vi "svx_Polar_Property_Change.vi"(0 "Property Name":string, 1 "Display State In":T2={"Property Name"=[], "Container bounds"={"Width"=550, "Height"=250}, "Scale range"={"Maximum"=1.0, "Increment"=1.0}, "PointIdx"=0, "Marker list"=[], "Color settings"={"Arrow color"=16860, "Magnitude major grid"=13816530, "Magnitude minor grid"=16777216, "Phase grid"=13816530, "Phase scale marker text"=0}, "Magnitude scale name"="Magnitude", "Magnitude scale format string"="%#.2e", "MagnitudeScale:Visible"=TRUE, "MagnitudeScaleLabel:Visible"=TRUE, "PhaseScale:Visible"=TRUE, "Marker:Visible"=TRUE, "Cursor:Visible"=FALSE, "CursorName:Visible"=TRUE, "Autoscale"=TRUE, "Marker color"=16860, "Line color"=16711680, "Cursor color"=16711680, "Magnitude scale marker color"=0, "Plot.Line Style"=0, "Plot.Line Width"=0, "Plot.Point Style"=0, "Cursor.Line Style"=0, "Cursor.Line Width"=0, "Cursor.Point Style"=0, "Cursor.Style"=4, "Marker.Point Style"=2, "Point/fill color"=16711680, "Background color"=16777225, "Cursor name"="", "Cursor Release"=refnum, "Scale Range Change"=refnum, "data size(s)"=[], "Selectors:Visible"=TRUE, "Selector:ring Strings"={"Selector:Custom Strings"=FALSE, "Selector:Row Strings []"=[], "Selector:Column Strings []"=[], "User:Row Strings []"=[], "User:Column Strings []"=[]}, "Lock Cursor Info Position"=FALSE, "CursLoc"={"magnitude"=0.0, "phase"=0.0, "time/rev/RPM"=0.0}, "Plot Area:Position"={"Left"=0, "Top"=0}, "Plot Area:Size"={"Width"=0, "Height"=0}, "Marker.Style"=0, "Indication Arcs"=[], "Arc.Selector"=0, "customized marker"=[], "tree Width"=0, " Parents Tags"=[], "Children Tags"=[], "open?"=[], "index"=[{"row index"=0, "column index"=0}], "Label"="", "custom strings changed"=FALSE, "Owning VI"=refnum, "Legend BG color"=16777225, "Legend font color"=0, "column Width"=203, "attribute"=variant} caption="State", 2 "data":T1, 5 "operation in":T5[](array[typedef]), 6 "Plot Legend":refnum<vi>, 7 "z scale graph":refnum<vi>, 8 "Polar Plot ref in":refnum<vi>, 9 "Cursor Info":refnum<vi>, 10 "Container Refnum":refnum<vi>) -> (15 "Display State Out":T2={"Property Name"=[], "Container bounds"={"Width"=550, "Height"=250}, "Scale range"={"Maximum"=1.0, "Increment"=1.0}, "PointIdx"=0, "Marker list"=[], "Color settings"={"Arrow color"=16860, "Magnitude major grid"=13816530, "Magnitude minor grid"=16777216, "Phase grid"=13816530, "Phase scale marker text"=0}, "Magnitude scale name"="Magnitude", "Magnitude scale format string"="%#.2e", "MagnitudeScale:Visible"=TRUE, "MagnitudeScaleLabel:Visible"=TRUE, "PhaseScale:Visible"=TRUE, "Marker:Visible"=TRUE, "Cursor:Visible"=FALSE, "CursorName:Visible"=TRUE, "Autoscale"=TRUE, "Marker color"=16860, "Line color"=16711680, "Cursor color"=16711680, "Magnitude scale marker color"=0, "Plot.Line Style"=0, "Plot.Line Width"=0, "Plot.Point Style"=0, "Cursor.Line Style"=0, "Cursor.Line Width"=0, "Cursor.Point Style"=0, "Cursor.Style"=4, "Marker.Point Style"=2, "Point/fill color"=16711680, "Background color"=16777225, "Cursor name"="", "Cursor Release"=refnum, "Scale Range Change"=refnum, "data size(s)"=[], "Selectors:Visible"=TRUE, "Selector:ring Strings"={"Selector:Custom Strings"=FALSE, "Selector:Row Strings []"=[], "Selector:Column Strings []"=[], "User:Row Strings []"=[], "User:Column Strings []"=[]}, "Lock Cursor Info Position"=FALSE, "CursLoc"={"magnitude"=0.0, "phase"=0.0, "time/rev/RPM"=0.0}, "Plot Area:Position"={"Left"=0, "Top"=0}, "Plot Area:Size"={"Width"=0, "Height"=0}, "Marker.Style"=0, "Indication Arcs"=[], "Arc.Selector"=0, "customized marker"=[], "tree Width"=0, " Parents Tags"=[], "Children Tags"=[], "open?"=[], "index"=[{"row index"=0, "column index"=0}], "Label"="", "custom strings changed"=FALSE, "Owning VI"=refnum, "Legend BG color"=16777225, "Legend font color"=0, "column Width"=203, "attribute"=variant} caption="State", 19 "operation out":T5[](array[typedef]))   [LabVIEW 2017, in "SVX Polar Plot.xctl"]
uses:
  <vilib>/addons/_XControls/Polar Plot/SVX Polar Plot.xctl
  <vilib>/addons/_XControls/Polar Plot/subVIs/svx_Polar_Plot_Internal_State.ctl
  <vilib>/addons/_XControls/Polar Plot/subVIs/svx_Polar_Indication_Arcs.ctl
  <vilib>/addons/_XControls/Polar Plot/subVIs/svx_Polar_Customized_Markers.ctl
  <vilib>/addons/_XControls/Polar Plot/subVIs/svx_Polar_Core_States.ctl
  <vilib>/Utility/miscctls.llb/LVAnnotationListTypeDef.ctl
  <vilib>/Utility/miscctls.llb/LVBoundsTypeDef.ctl
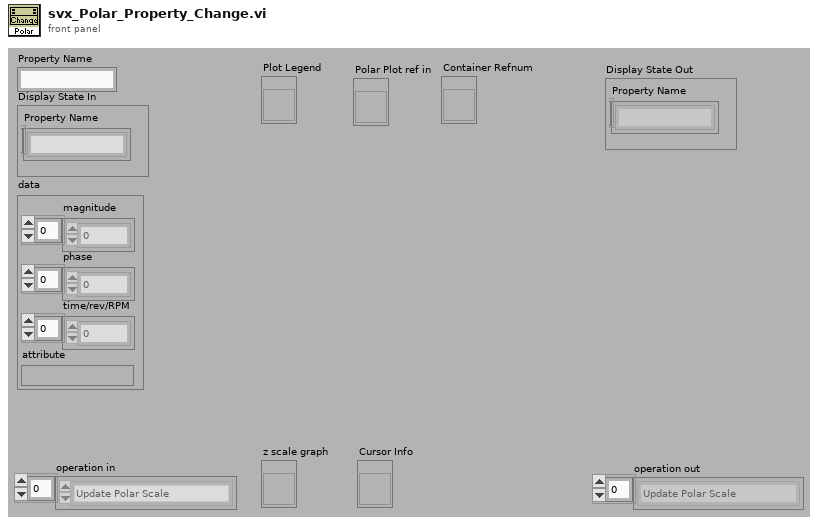
[diagram p1: front panel]
types:
  T1 = cluster{"magnitude":dbl[], "phase":dbl[], "time/rev/RPM":dbl[], "attribute":variant}
  T2 = typedef "SVX Polar Plot.xctl/svx_Polar_Plot_Internal_State.ctl" = cluster{"Property Name":string[], "Container bounds":cluster{"Width":u32, "Height":u32}, "Scale range":cluster{"Maximum":dbl, "Increment":dbl}, "PointIdx":i32, "Marker list":cluster{"Name":string, "Color":u32, "Style":u8, "Point Style":u8, "Name Visible":bool, "Allow Drag":bool, "Annotation Mode":u32, "Plot":i32, "Index":i32, "Position":cluster{"X":dbl, "Y":dbl}, "X Scale":u32, "Y Scale":u32, "Show Arrow":bool, "Lock Name":bool, "Plot Area":i32, "Label Offset":cluster{"X":dbl, "Y":dbl}}[], "Color settings":cluster{"Arrow color":u32, "Magnitude major grid":u32, "Magnitude minor grid":u32, "Phase grid":u32, "Phase scale marker text":u32}, "Magnitude scale name":string, "Magnitude scale format string":string, "MagnitudeScale:Visible":bool, "MagnitudeScaleLabel:Visible":bool, "PhaseScale:Visible":bool, "Marker:Visible":bool, "Cursor:Visible":bool, "CursorName:Visible":bool, "Autoscale":bool, "Marker color":u32, "Line color":u32, "Cursor color":u32, "Magnitude scale marker color":u32, "Plot.Line Style":i32, "Plot.Line Width":i32, "Plot.Point Style":i32, "Cursor.Line Style":i32, "Cursor.Line Width":i32, "Cursor.Point Style":i32, "Cursor.Style":i32, "Marker.Point Style":i32, "Point/fill color":u32, "Background color":u32, "Cursor name":string, "Cursor Release":refnum<user-event>, "Scale Range Change":refnum<user-event>, "data size(s)":i32[], "Selectors:Visible":bool, "Selector:ring Strings":cluster{"Selector:Custom Strings":bool, "Selector:Row Strings []":string[], "Selector:Column Strings []":string[], "User:Row Strings []":string[], "User:Column Strings []":string[]}, "Lock Cursor Info Position":bool, "CursLoc":cluster{"magnitude":dbl, "phase":dbl, "time/rev/RPM":dbl}, "Plot Area:Position":cluster{"Left":i32, "Top":i32}, "Plot Area:Size":cluster{"Width":u32, "Height":u32}, "Marker.Style":i32, "Indication Arcs":T3, "Arc.Selector":u16, "customized marker":T4, "tree Width":u32, " Parents Tags":string[], "Children Tags":string[], "open?":bool[], "index":cluster{"row index":i32, "column index":i32}[], "Label":string, "custom strings changed":bool, "Owning VI":refnum<vi>, "Legend BG color":u32, "Legend font color":u32, "column Width":u32, "attribute":variant}
  T3 = typedef "SVX Polar Plot.xctl/svx_Polar_Indication_Arcs.ctl" = cluster{"Name":string, "Start radius":dbl, "End radius":dbl, "Line Style":i32, "Line Width":i32, "Border color":u32, "Fill color":u32, "Start angle":i16, "End angle":i16, "Visible":bool}[]
  T4 = typedef "SVX Polar Plot.xctl/svx_Polar_Customized_Markers.ctl" = cluster{"Name":string, "Color":u32, "Style":u8, "Point Style":u8, "Name Visible":bool, "Allow Drag":bool, "Annotation Mode":u32, "Plot":i32, "Index":i32, "Position":cluster{"Magnitude":dbl, "Phase":dbl}, "X Scale":u32, "Y Scale":u32, "Show Arrow":bool, "Lock Name":bool, "Plot Area":i32, "Label Offset":cluster{"Magnitude":dbl, "Phase":dbl}}[]
  T5 = typedef "SVX Polar Plot.xctl/svx_Polar_Core_States.ctl" = enum16{"Update Polar Scale", "Cursor Release", "Autoscale", "Update Annotation", "Force Update Polar Scale", "Update Data", "Update Tree String", "Update Tree Checkbox", "Update Tree Opening", "Change Minimum Size"}
  T6 = typedef "LVAnnotationListTypeDef.ctl" = cluster{"Name":string, "Color":u32, "Style":u8, "Point Style":u8, "Name Visible":bool, "Allow Drag":bool, "Annotation Mode":u32, "Plot":i32, "Index":i32, "Position":cluster{"X":dbl, "Y":dbl}, "X Scale":u32, "Y Scale":u32, "Show Arrow":bool, "Lock Name":bool, "Plot Area":i32, "Label Offset":cluster{"X":dbl, "Y":dbl}}[]
  T7 = typedef "LVBoundsTypeDef.ctl" = cluster{"Width":u32, "Height":u32}
  T8 = typedef "LVCursorListTypeDef.ctl" = cluster{"Name":string, "Color":u32, "Style":u8, "Point Style":u8, "Name Visible":bool, "Allow Drag":bool, "Cursor Mode":u32, "Plot":i32, "Index":i32, "Position":cluster{"X":dbl, "Y":dbl}, "X Scale":u32, "Y Scale":u32, "Watch Plots":i32[], "Watch All Plots":bool, "Plot Area":i32, "Label Offset":cluster{"X":dbl, "Y":dbl}}[]
  T9 = cluster{"Name":string, "Color":u32, "Style":u8, "Point Style":u8, "Name Visible":bool, "Allow Drag":bool, "Cursor Mode":u32, "Plot":i32, "Index":i32, "Position":cluster{"X":dbl, "Y":dbl}, "X Scale":u32, "Y Scale":u32, "Watch Plots":i32[], "Watch All Plots":bool, "Plot Area":i32, "Label Offset":cluster{"X":dbl, "Y":dbl}}
  T10 = cluster{"Arrow color":u32, "Magnitude major grid":u32, "Magnitude minor grid":u32, "Phase grid":u32, "Phase scale marker text":u32}
  T11 = cluster{"Name":string, "Color":u32, "Style":u8, "Point Style":u8, "Name Visible":bool, "Allow Drag":bool, "Annotation Mode":u32, "Plot":i32, "Index":i32, "Position":cluster{"X":dbl, "Y":dbl}, "X Scale":u32, "Y Scale":u32, "Show Arrow":bool, "Lock Name":bool, "Plot Area":i32, "Label Offset":cluster{"X":dbl, "Y":dbl}}[]
  T12 = cluster{"Name":string, "Color":u32, "Style":u8, "Point Style":u8, "Name Visible":bool, "Allow Drag":bool, "Annotation Mode":u32, "Plot":i32, "Index":i32, "Position":cluster{"X":dbl, "Y":dbl}, "X Scale":u32, "Y Scale":u32, "Show Arrow":bool, "Lock Name":bool, "Plot Area":i32, "Label Offset":cluster{"X":dbl, "Y":dbl}}
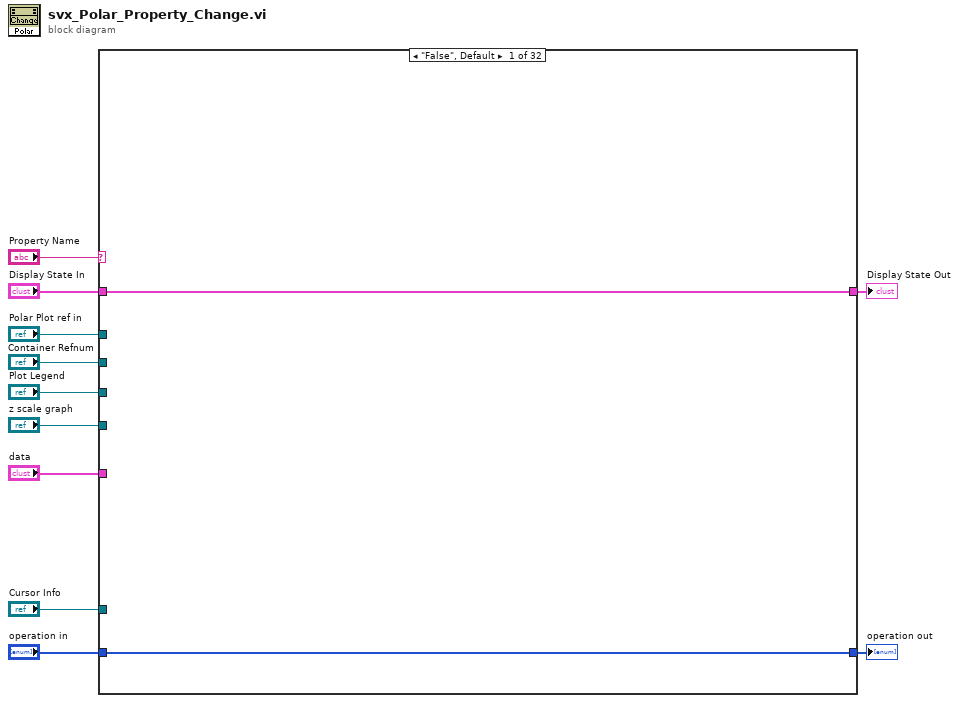
[diagram p0: block diagram]
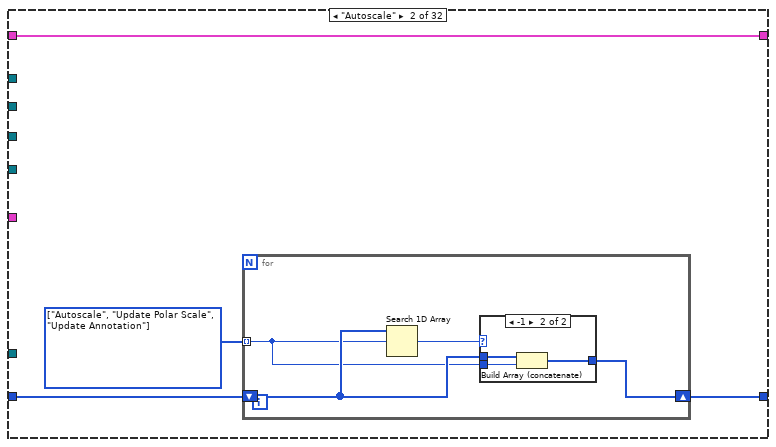
[diagram p2: hidden frame]
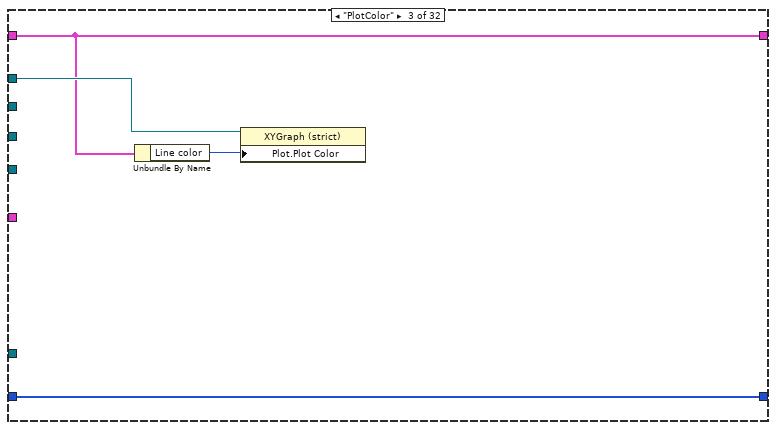
[diagram p4: hidden frame]
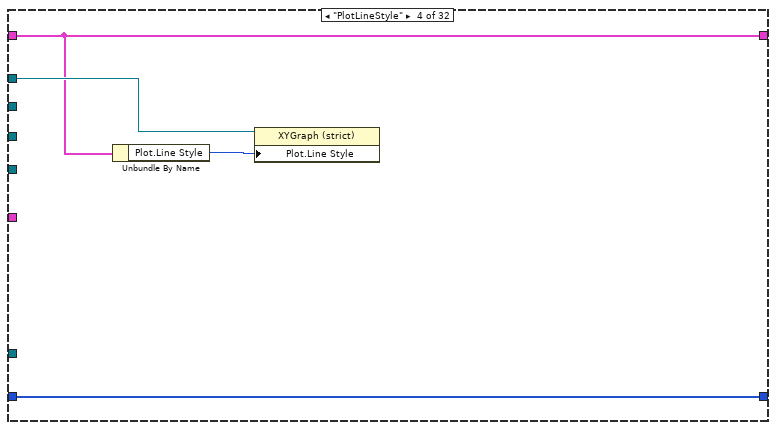
[diagram p5: hidden frame]
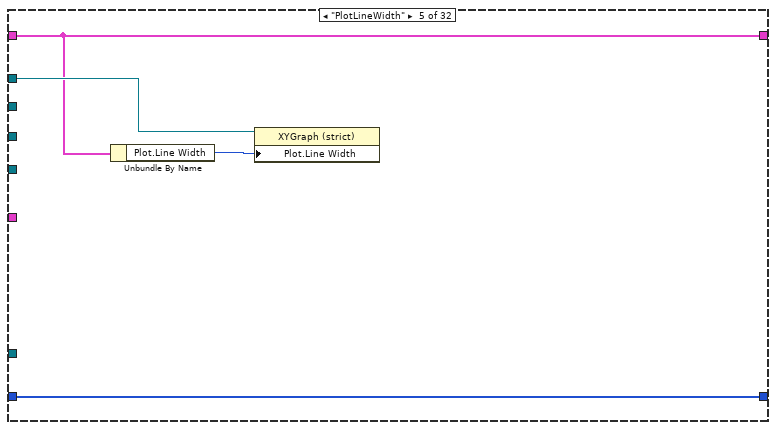
[diagram p6: hidden frame]
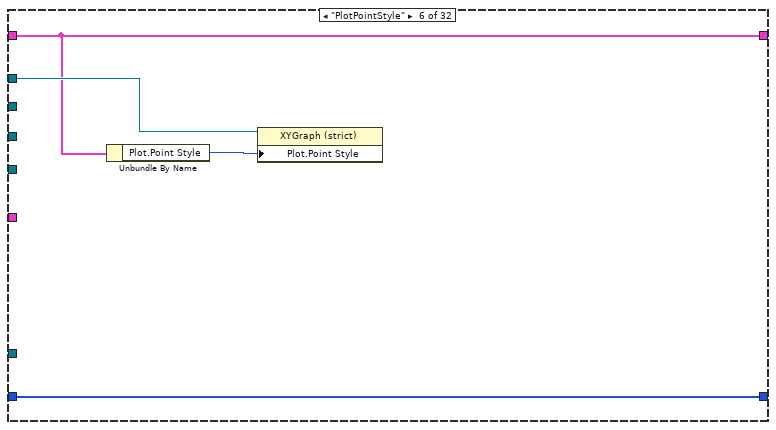
[diagram p7: hidden frame]
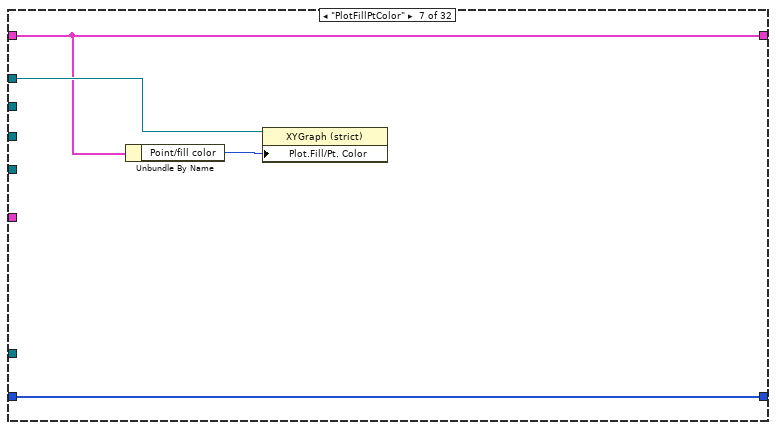
[diagram p8: hidden frame]
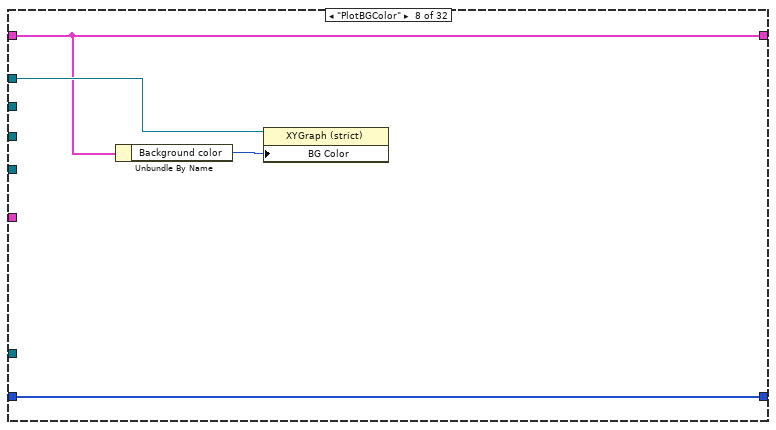
[diagram p9: hidden frame]
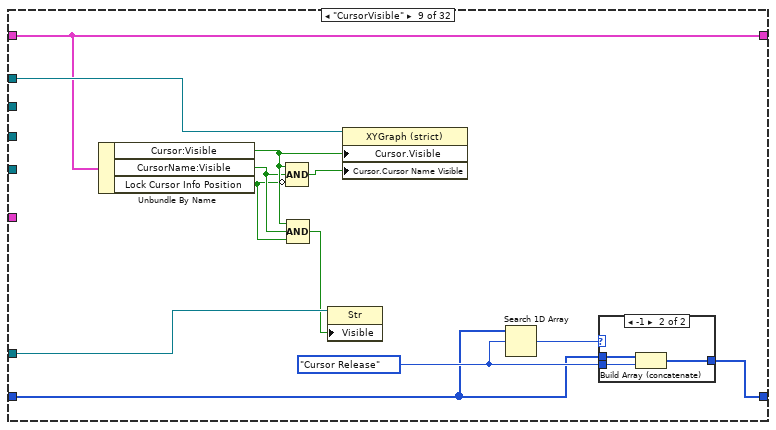
[diagram p10: hidden frame]
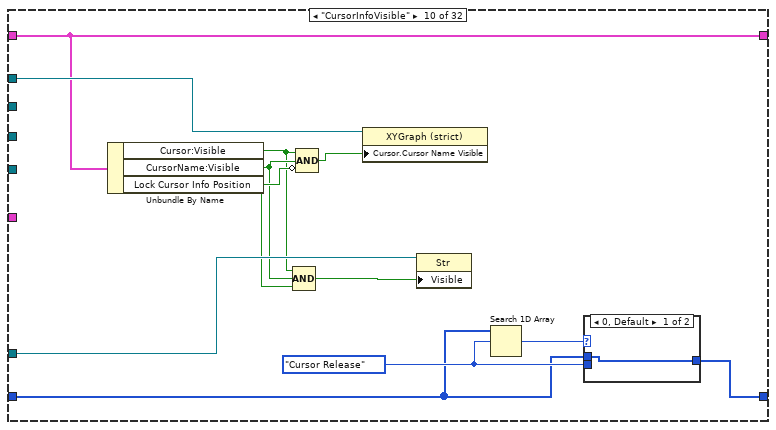
[diagram p12: hidden frame]
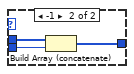
[diagram p13: hidden frame]
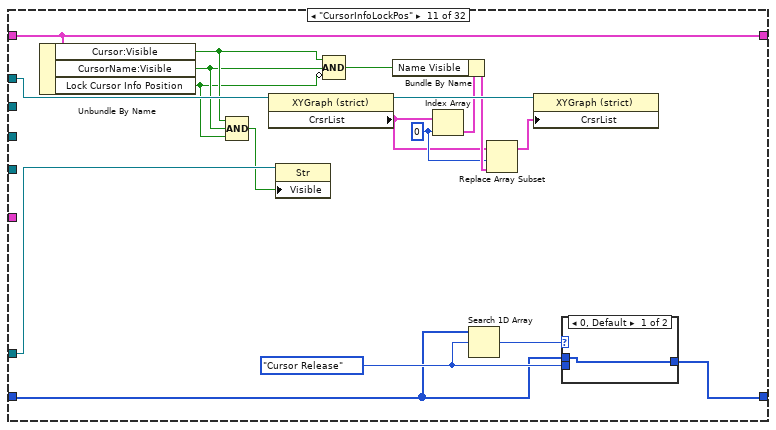
[diagram p14: hidden frame]
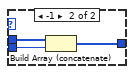
[diagram p15: hidden frame]
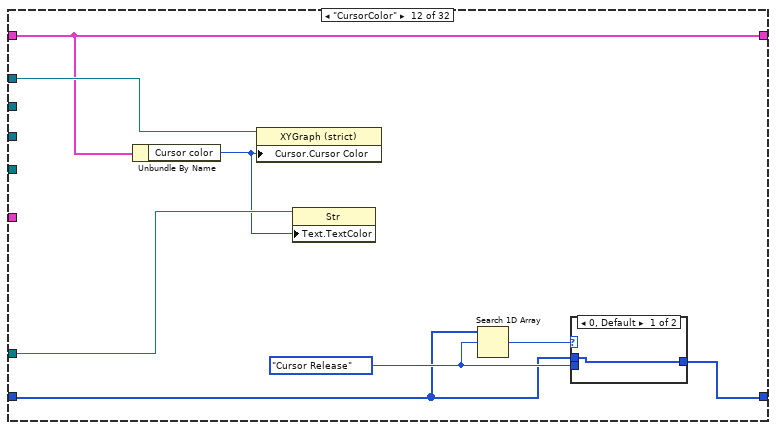
[diagram p16: hidden frame]
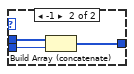
[diagram p17: hidden frame]
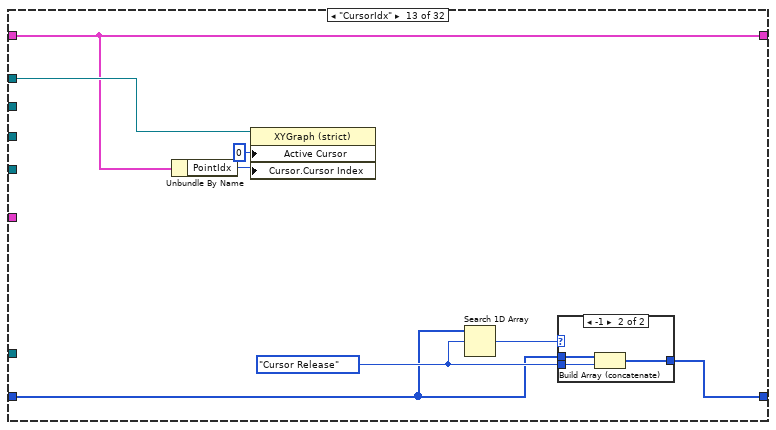
[diagram p18: hidden frame]
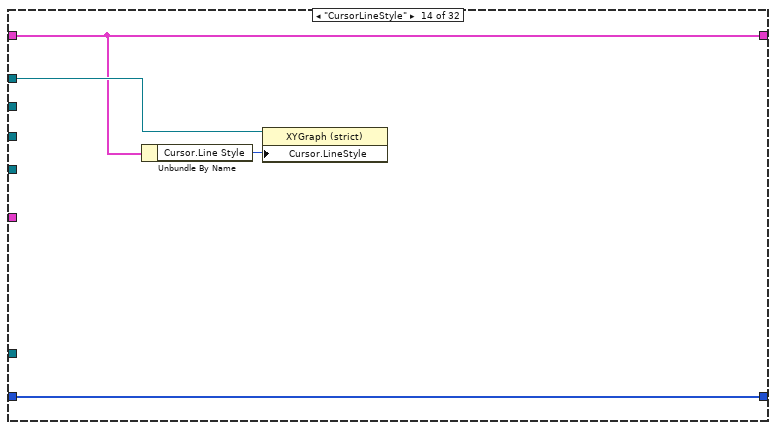
[diagram p20: hidden frame]
diagram:
  n1 = case shown="\"False\", Default" "Property Name" {
    tunnel: "Display State In" -> [w12 w16 w26 w30 w34 w38 w42 w46 w60 w76 w99 w110 w122 w128 w132 w136 w140 w144 w166 w176 w180 w188 w197 w207 w221 w230 w265 w279 w290 w303 w308 w312]
    tunnel: "operation in" -> [w13 w15 w29 w33 w37 w41 w45 w49 w50 w67 w88 w104 w116 w131 w135 w139 w143 w145 w167 w177 w181 w190 w193 w206 w223 w226 w263 w273 w284 w307 _ w315]
    tunnel: [w13 w17 w29 w33 w37 w41 w45 w49 w51 w66 w87 w105 w117 w131 w135 w139 w143 w145 w167 w177 w181 w190 w194 w204 w223 w226 w263 w273 w284 w305 w309 w315] -> w8
    tunnel: "Polar Plot ref in" -> [_ _ w28 w32 w36 w40 w44 w48 w61 w77 w92 w111 w123 w130 w134 w138 w142 w148 w170 _ _ w187 _ w212 w222 w229 w262 w274 w285 w301 _ _]
    tunnel: "z scale graph" -> [_ _ _ _ _ _ _ _ _ _ _ _ _ _ _ _ _ w147 w169 w179 w183 w186 w199 w211 _ w224 _ _ _ w299 _ _]
    tunnel: "data" -> [_ _ _ _ _ _ _ _ _ _ _ _ _ _ _ _ _ _ w165 _ _ _ _ _ _ w228 _ _ _ _ _ _]
    tunnel: [w12 w16 w26 w30 w34 w38 w42 w46 w60 w76 w99 w110 w122 w128 w132 w136 w140 w144 w166 w176 w180 w188 w197 w207 w221 w227 w264 w275 w286 w304 w308 w312] -> w6
    tunnel: "Cursor Info" -> [_ _ _ _ _ _ _ _ w59 w74 w91 w109 _ _ _ _ _ _ _ _ _ _ _ _ _ _ _ _ _ _ _ _]
    tunnel: "Plot Legend" -> [_ _ _ _ _ _ _ _ _ _ _ _ _ _ _ _ _ _ _ _ _ _ _ _ _ _ _ _ _ w300 _ w314]
    tunnel: "Container Refnum" -> [_ _ _ _ _ _ _ _ _ _ _ _ _ _ _ _ _ _ _ _ _ _ _ _ _ _ _ _ _ w302 _ _]
    frame "False", Default {
    }
    frame "Autoscale" {
      w14 = T5[] [enum."Autoscale", enum."Update Polar Scale", enum."Update Annotation"] items=["Update Polar Scale", "Cursor Release", "Autoscale", "Update Annotation", "Force Update Polar Scale", "Update Data", "Update Tree String", "Update Tree Checkbox", "Update Tree Opening", "Change Minimum Size"]
      n2 = for {
        shift-right: [w21] -> w17
        shift-left: w15 -> [w20]
        tunnel: w14 -> [w18] mode=indexing
        n3 = Search 1D Array(1D array=w20, element=w18) -> (index of element=w19:i32)  [unwired: 1 in]
        n4 = case shown="-1" w19 {
          tunnel: [w22 w25] -> w21
          tunnel: w20 -> [w22 w24]
          tunnel: w18 -> [_ w23]
          frame 0, Default {
          }
          frame -1 {
            n5 = Build Array (concatenate)(w24, w23) -> (w25:T5[])
          }
        }
      }
    }
    frame "PlotColor" {
      n6 = Unbundle By Name(w26) -> ("Line color"=w27:u32)
      n7 = property class="XYGraph (strict)"(reference=w28, "Plot.Plot Color"=w27) -> ()  [unwired: 1 in, 2 out]
    }
    frame "PlotLineStyle" {
      n8 = Unbundle By Name(w30) -> ("Plot.Line Style"=w31:i32)
      n9 = property class="XYGraph (strict)"(reference=w32, "Plot.Line Style"=w31) -> ()  [unwired: 1 in, 2 out]
    }
    frame "PlotLineWidth" {
      n10 = Unbundle By Name(w34) -> ("Plot.Line Width"=w35:i32)
      n11 = property class="XYGraph (strict)"(reference=w36, "Plot.Line Width"=w35) -> ()  [unwired: 1 in, 2 out]
    }
    frame "PlotPointStyle" {
      n12 = Unbundle By Name(w38) -> ("Plot.Point Style"=w39:i32)
      n13 = property class="XYGraph (strict)"(reference=w40, "Plot.Point Style"=w39) -> ()  [unwired: 1 in, 2 out]
    }
    frame "PlotFillPtColor" {
      n14 = Unbundle By Name(w42) -> ("Point/fill color"=w43:u32)
      n15 = property class="XYGraph (strict)"(reference=w44, "Plot.Fill/Pt. Color"=w43) -> ()  [unwired: 1 in, 2 out]
    }
    frame "PlotBGColor" {
      n16 = Unbundle By Name(w46) -> ("Background color"=w47:u32)
      n17 = property class="XYGraph (strict)"(reference=w48, "BG Color"=w47) -> ()  [unwired: 1 in, 2 out]
    }
    frame "CursorVisible" {
      w52 = svx_Polar_Core_States."Cursor Release" ("svx_Polar_Core_States")
      n18 = Unbundle By Name(w60) -> ("Cursor:Visible"=w57:bool, "CursorName:Visible"=w56:bool, "Lock Cursor Info Position"=w55:bool)
      n19 = Compound Arithmetic op=AND(w57, w56, invert w55) -> (w58:bool)
      n20 = Compound Arithmetic op=AND(w57, w56, w55) -> (w54:bool)
      n21 = property class="Str"(reference=w59, "Visible"=w54) -> ()  [unwired: 1 in, 2 out]
      n22 = property class="XYGraph (strict)"(reference=w61, "Cursor.Visible"=w57, "Cursor.Cursor Name Visible"=w58) -> ()  [unwired: 1 in, 2 out]
      n23 = Search 1D Array(1D array=w50, element=w52) -> (index of element=w53:i32)  [unwired: 1 in]
      n24 = case shown="-1" w53 {
        tunnel: [w62 w65] -> w51
        tunnel: w50 -> [w62 w64]
        tunnel: w52 -> [_ w63]
        frame 0, Default {
        }
        frame -1 {
          n25 = Build Array (concatenate)(w64, w63) -> (w65:T5[])
        }
      }
    }
    frame "CursorInfoVisible" {
      w68 = svx_Polar_Core_States."Cursor Release" ("svx_Polar_Core_States")
      n26 = Unbundle By Name(w76) -> ("Cursor:Visible"=w71:bool, "CursorName:Visible"=w72:bool, "Lock Cursor Info Position"=w73:bool)
      n27 = Compound Arithmetic op=AND(w71, w72, w73) -> (w70:bool)
      n28 = Compound Arithmetic op=AND(w71, w72, invert w73) -> (w75:bool)
      n29 = property class="XYGraph (strict)"(reference=w77, "Cursor.Cursor Name Visible"=w75) -> ()  [unwired: 1 in, 2 out]
      n30 = property class="Str"(reference=w74, "Visible"=w70) -> ()  [unwired: 1 in, 2 out]
      n31 = Search 1D Array(1D array=w67, element=w68) -> (index of element=w69:i32)  [unwired: 1 in]
      n32 = case shown="0, Default" w69 {
        tunnel: [w78 w81] -> w66
        tunnel: w67 -> [w78 w80]
        tunnel: w68 -> [_ w79]
        frame 0, Default {
        }
        frame -1 {
          n33 = Build Array (concatenate)(w80, w79) -> (w81:T5[])
        }
      }
    }
    frame "CursorInfoLockPos" {
      w89 = svx_Polar_Core_States."Cursor Release" ("svx_Polar_Core_States")
      w95 = 0 ("index")
      n34 = Unbundle By Name(w99) -> ("Cursor:Visible"=w85:bool, "CursorName:Visible"=w84:bool, "Lock Cursor Info Position"=w83:bool)
      n35 = Compound Arithmetic op=AND(w85, w84, w83) -> (w82:bool)
      n36 = property class="XYGraph (strict)"(reference=w92) -> (reference out=w97:refnum<vi>, "CrsrList"=w94:T8)  [unwired: 1 in, 1 out]
      n37 = property class="Str"(reference=w91, "Visible"=w82) -> ()  [unwired: 1 in, 2 out]
      n38 = Compound Arithmetic op=AND(w85, w84, invert w83) -> (w86:bool)
      n39 = Index Array(array=w94, index=w95) -> (element=w93:T9)
      n40 = Bundle By Name(cluster=w93, "Name Visible"=w86) -> (w96:T9)
      n41 = Search 1D Array(1D array=w88, element=w89) -> (index of element=w90:i32)  [unwired: 1 in]
      n42 = Replace Array Subset(array=w94, new element=w96, index=w95) -> (w98:T8)
      n43 = property class="XYGraph (strict)"(reference=w97, "CrsrList"=w98) -> ()  [unwired: 1 in, 2 out]
      n44 = case shown="0, Default" w90 {
        tunnel: [w100 w103] -> w87
        tunnel: w88 -> [w100 w102]
        tunnel: w89 -> [_ w101]
        frame 0, Default {
        }
        frame -1 {
          n45 = Build Array (concatenate)(w102, w101) -> (w103:T5[])
        }
      }
    }
    frame "CursorColor" {
      w106 = svx_Polar_Core_States."Cursor Release" ("svx_Polar_Core_States")
      n46 = Unbundle By Name(w110) -> ("Cursor color"=w108:u32)
      n47 = property class="XYGraph (strict)"(reference=w111, "Cursor.Cursor Color"=w108) -> ()  [unwired: 1 in, 2 out]
      n48 = property class="Str"(reference=w109, "Text.TextColor"=w108) -> ()  [unwired: 1 in, 2 out]
      n49 = Search 1D Array(1D array=w104, element=w106) -> (index of element=w107:i32)  [unwired: 1 in]
      n50 = case shown="0, Default" w107 {
        tunnel: [w112 w115] -> w105
        tunnel: w104 -> [w112 w114]
        tunnel: w106 -> [_ w113]
        frame 0, Default {
        }
        frame -1 {
          n51 = Build Array (concatenate)(w114, w113) -> (w115:T5[])
        }
      }
    }
    frame "CursorIdx" {
      w118 = svx_Polar_Core_States."Cursor Release" ("svx_Polar_Core_States")
      n52 = Unbundle By Name(w122) -> ("PointIdx"=w120:i32)
      n53 = property class="XYGraph (strict)"(reference=w123, "Active Cursor"=u32 0, "Cursor.Cursor Index"=w120) -> ()  [unwired: 1 in, 2 out]
      n54 = Search 1D Array(1D array=w116, element=w118) -> (index of element=w119:i32)  [unwired: 1 in]
      n55 = case shown="-1" w119 {
        tunnel: [w124 w127] -> w117
        tunnel: w116 -> [w124 w126]
        tunnel: w118 -> [_ w125]
        frame 0, Default {
        }
        frame -1 {
          n56 = Build Array (concatenate)(w126, w125) -> (w127:T5[])
        }
      }
    }
    frame "CursorLineStyle" {
      n57 = Unbundle By Name(w128) -> ("Cursor.Line Style"=w129:i32)
      n58 = property class="XYGraph (strict)"(reference=w130, "Cursor.LineStyle"=w129) -> ()  [unwired: 1 in, 2 out]
    }
    frame "CursorLineWidth" {
      n59 = Unbundle By Name(w132) -> ("Cursor.Line Width"=w133:i32)
      n60 = property class="XYGraph (strict)"(reference=w134, "Cursor.LineWidth"=w133) -> ()  [unwired: 1 in, 2 out]
    }
    frame "CursorPointStyle" {
      n61 = Unbundle By Name(w136) -> ("Cursor.Point Style"=w137:i32)
      n62 = property class="XYGraph (strict)"(reference=w138, "Cursor.Cursor Point Style"=w137) -> ()  [unwired: 1 in, 2 out]
    }
    frame "CursorStyle" {
      n63 = Unbundle By Name(w140) -> ("Cursor.Style"=w141:i32)
      n64 = property class="XYGraph (strict)"(reference=w142, "Cursor.Cursor Style"=w141) -> ()  [unwired: 1 in, 2 out]
    }
    frame "MagnitudeScaleVisible" {
      n65 = Unbundle By Name(w144) -> ("MagnitudeScale:Visible"=w146:bool)
      n66 = case shown="True" w146 {
        tunnel: w148 -> [w151 w159]
        tunnel: w147 -> [w149 w158]
        frame False {
          n67 = property on="Property Node" class="XYGraph (strict)"(reference=w151) -> (reference out=w150:refnum<vi>, "Left"=w157:i32, "Top"=w155:i32)  [unwired: 1 in, 1 out]
          n68 = property on="Property Node" class="XYGraph (strict)"(reference=w150) -> ("Width"=w156:u32, "Height"=w154:u32)  [unwired: 1 in, 2 out]
          n69 = Subtract(x=w157, y=w156) -> (x-y=w153:u32)
          n70 = Subtract(x=w155, y=w154) -> (x-y=w152:u32)
          n71 = property on="Property Node" class="XYGraph (strict)"(reference=w149, "Left"=w153, "Top"=w152) -> ()  [unwired: 1 in, 2 out]
        }
        frame True {
          n72 = call <vilib>:"svx_Polar_Align_Plot_Area.vi"("z scale graph ref in"=w158, "Polar Plot ref in"=w159) -> ()  [unwired: 8 in, 2 out]
        }
      }
    }
    frame "IndicationArcsChanged", "MagnitudeMajorGridColor", "MagnitudeMinorGridColor", "PhaseScaleColor", "PhaseScaleTextColor", "PhaseScaleVisible", "PlotArrowColor" {
      n73 = Unbundle By Name(w166) -> ("MagnitudeScale:Visible"=w171:bool, "PhaseScale:Visible"=w175:bool, "Color settings"=w174:T10, "Color settings.Magnitude major grid"=w168:u32, "Indication Arcs"=w161:T3, "Background color"=w160:u32)
      n74 = property class="XYGraph (strict)"(reference=w169, "YScale.MinorTickColor"=w168, "YScale.TickColor"=w168) -> (reference out=w172:refnum<vi>)  [unwired: 1 in, 1 out]
      n75 = call <vilib>:"svx_Polar_Read_Attribute.vi"("polar plot"=w165) -> ("is OA Polar Plot?"=w163:bool, "shaft rotating direction"=w164:u16, "probe angle [deg]"=w162:u16)  [unwired: 13 in, 3 out]
      n76 = call <vilib>:"svx_Polar_Draw_Scale.vi"("horizontal line visible"=w171, "thetaScale visible"=w175, "draw rotating direct"=w163, "color settings"=w174, "z scale graph ref in"=w172, "shaft rotating direction"=w164, "Polar Plot ref in"=w170, "probe angle [deg]"=w162, "Indication Arcs"=w161, "Background color"=w160) -> ("new picture"=w173:picture)  [unwired: 9 in]
      n77 = property class="XYGraph (strict)"(reference=w170, "PlotImages.Middle"=w173) -> ()  [unwired: 1 in, 2 out]
    }
    frame "MagnitudeScaleTextColor" {
      n78 = Unbundle By Name(w176) -> ("Magnitude scale marker color"=w178:u32)
      n79 = property class="XYGraph (strict)"(reference=w179, "YScale.Text Color"=w178) -> ()  [unwired: 1 in, 2 out]
    }
    frame "MagnitudeScaleLableText" {
      n80 = Unbundle By Name(w180) -> ("Magnitude scale name"=w182:string)
      n81 = property class="XYGraph (strict)"(reference=w183, "YScale.NameLbl.Text"=w182) -> ()  [unwired: 1 in, 2 out]
    }
    frame "MagnitudeScaleLableVisible" {
      n82 = Unbundle By Name(w188) -> ("MagnitudeScaleLabel:Visible"=w185:bool, "MagnitudeScale:Visible"=w184:bool)
      n83 = property class="XYGraph (strict)"(reference=w186, "YScale.NameLbl.Visible"=w185) -> (reference out=w189:refnum<vi>)  [unwired: 1 in, 1 out]
      n84 = case shown="True" w184 {
        tunnel: w189 -> [_ w192]
        tunnel: w187 -> [_ w191]
        frame False {
        }
        frame True {
          n85 = call <vilib>:"svx_Polar_Align_Plot_Area.vi"("z scale graph ref in"=w192, "Polar Plot ref in"=w191) -> ()  [unwired: 8 in, 2 out]
        }
      }
    }
    frame "MagnitudeScaleFormatString" {
      w195 = svx_Polar_Core_States."Update Polar Scale" ("svx_Polar_Core_States")
      n86 = Unbundle By Name(w197) -> ("Magnitude scale format string"=w198:string)
      n87 = property class="XYGraph (strict)"(reference=w199, "YScale.FormatString"=w198) -> ()  [unwired: 1 in, 2 out]
      n88 = Search 1D Array(1D array=w193, element=w195) -> (index of element=w196:i32)  [unwired: 1 in]
      n89 = case shown="-1" w196 {
        tunnel: [w200 w203] -> w194
        tunnel: w193 -> [w200 w202]
        tunnel: w195 -> [_ w201]
        frame 0, Default {
        }
        frame -1 {
          n90 = Build Array (concatenate)(w202, w201) -> (w203:T5[])
        }
      }
    }
    frame "MagnitudeScaleRangeMaximum" {
      w205 = T5[] [enum."Update Polar Scale", enum."Update Annotation"] items=["Update Polar Scale", "Cursor Release", "Autoscale", "Update Annotation", "Force Update Polar Scale", "Update Data", "Update Tree String", "Update Tree Checkbox", "Update Tree Opening", "Change Minimum Size"]
      n91 = Unbundle By Name(w207) -> ("Scale range.Maximum"=w210:dbl)
      n92 = Negate(x=w210) -> (-x=w216:dbl)
      n93 = property on="Property Node" class="XYGraph (strict)"(reference=w212, "XScale.Maximum"=w210, "XScale.Minimum"=w216, "YScale.Maximum"=w210, "YScale.Minimum"=w216) -> (reference out=w209:refnum<vi>, error out=w213:errorcluster)  [unwired: 1 in]
      n94 = property on="Property Node" class="XYGraph (strict)"(reference=w211, error in=w213, "YScale.Flipped"=FALSE ("Y Scale.Flipped"), "YScale.Maximum"=w210, "YScale.Minimum"=0.0 ("Minimum")) -> (reference out=w208:refnum<vi>)  [unwired: 1 out]
      n95 = Build Array (concatenate)(w206, w205) -> (w204:T5[])
      n96 = call <vilib>:"svx_Polar_Align_Plot_Area.vi"("z scale graph ref in"=w208, "Polar Plot ref in"=w209) -> ()  [unwired: 8 in, 2 out]
    }
    frame "MarkerList" {
      n97 = Unbundle By Name(w221) -> ("Marker list"=w220:T11)
      n98 = property on="Property Node" class="XYGraph (strict)"(reference=w222, "AnntList"=w220) -> (reference out=w219:refnum<vi>)  [unwired: 1 in, 1 out]
      n99 = property on="Property Node" class="XYGraph (strict)"(reference=w219) -> (reference out=w218:refnum<vi>, "AnntList"=w217:T6)  [unwired: 1 in, 1 out]
      n100 = property on="Property Node" class="XYGraph (strict)"(reference=w218, "AnntList"=w217) -> ()  [unwired: 1 in, 2 out]
    }
    frame "MarkerVisible" {
      n101 = Unbundle By Name(w230) -> ("Marker:Visible"=w231:bool, "customized marker"=w225:T4)
      n102 = case shown="False" w231 {
        selector: w231 -> [w241 _]
        tunnel: w230 -> [w242 w250]
        tunnel: w229 -> [w232 w256]
        tunnel: w228 -> [w233 w244]
        tunnel: [w240 w251] -> w227
        tunnel: w225 -> [w238 w248]
        tunnel: w224 -> [_ _]
        frame False {
          n103 = call <vilib>:"svx_Polar_Convert_CustomizedMarkers.vi"("polar plot"=w233, "customized marker"=w238) -> ("customized annotations"=w237:T6)  [unwired: 9 in]
          n104 = property class="XYGraph (strict)"(reference=w232, "AnntList"=w237) -> (reference out=w234:refnum<vi>)  [unwired: 1 in, 1 out]
          n105 = property class="XYGraph (strict)"(reference=w234) -> (reference out=w236:refnum<vi>, "AnntList"=w235:T6)  [unwired: 1 in, 1 out]
          n106 = Bundle By Name(cluster=w242, "Marker:Visible"=w241, "Marker list"=T6 [] ("Annotation List")) -> (w240:T2)
          n107 = property class="XYGraph (strict)"(reference=w236, "AnntList"=w235) -> ()  [unwired: 1 in, 2 out]
        }
        frame True {
          # "Do NOT remove this Read/Write operations.\nIt's not redundant. It is used to solve a update problem."
          n108 = call <vilib>:"svx_Polar_Read_Attribute.vi"("polar plot"=w244) -> ("reference label"=w249:u16)  [unwired: 13 in, 5 out]
          n109 = call <vilib>:"svx_Polar_Get_Annotation.vi"("Polar Plot"=w256, "data"=w244) -> ("Array"=w257:cluster{dbl, dbl}[], "marker value"=w258:dbl[])  [unwired: 8 in]
          n110 = case shown="1, Default" w249 {
            tunnel: [i16 2 ("precision (6)") i16 0 ("precision (6)")] -> w259
            frame 0 {
            }
            frame 1, Default {
            }
          }
          n111 = call <vilib>:"svx_Polar_Draw_Annotation.vi"("Polar Plot ref in"=w256, "State in"=w250, "position array"=w257, "Annotation Values"=w258, "precision (6)"=w259) -> ("State out"=w253:T2, "Polar Plot ref out"=w243:refnum<vi>, "AnntList"=w245:T6)  [unwired: 8 in]
          n112 = call <vilib>:"svx_Polar_Convert_CustomizedMarkers.vi"("polar plot"=w244, "customized marker"=w248) -> ("customized annotations"=w247:T6)  [unwired: 9 in]
          n113 = Build Array (concatenate)(w245, w247) -> (w246:T6)
          n114 = property class="XYGraph (strict)"(reference=w243, "AnntList"=w246) -> (reference out=w255:refnum<vi>)  [unwired: 1 in, 1 out]
          n115 = property class="XYGraph (strict)"(reference=w255) -> (reference out=w254:refnum<vi>, "AnntList"=w252:T6)  [unwired: 1 in, 1 out]
          n116 = property class="XYGraph (strict)"(reference=w254, "AnntList"=w252) -> ()  [unwired: 1 in, 2 out]
          n117 = Bundle By Name(cluster=w253, "Marker list"=w245) -> (w251:T2)
        }
      }
    }
    frame "MarkerColor" {
      n118 = Unbundle By Name(w265) -> ("Marker color"=w266:u32)
      n119 = property class="XYGraph (strict)"(reference=w262) -> (reference out=w269:refnum<vi>, "AnntList"=w268:T6)  [unwired: 1 in, 1 out]
      n120 = for {
        tunnel: w268 -> [w272] mode=indexing
        tunnel: w266 -> [w271]
        tunnel: [w270] -> w267 mode=indexing
        n121 = Bundle By Name(cluster=w272, "Color"=w271) -> (w270:T12)
      }
      n122 = property class="XYGraph (strict)"(reference=w269, "AnntList"=w267) -> ()  [unwired: 1 in, 2 out]
      n123 = Bundle By Name(cluster=w265, "Marker list"=w267) -> (w264:T2)
    }
    frame "MarkerPtStyle" {
      n124 = property class="XYGraph (strict)"(reference=w274) -> (reference out=w280:refnum<vi>, "AnntList"=w277:T6)  [unwired: 1 in, 1 out]
      n125 = Unbundle By Name(w279) -> ("Marker.Point Style"=w278:i32)
      n126 = for {
        tunnel: w278 -> [w283]
        tunnel: w277 -> [w282] mode=indexing
        tunnel: [w281] -> w276 mode=indexing
        n127 = Bundle By Name(cluster=w282, "Point Style"=w283) -> (w281:T12)
      }
      n128 = Bundle By Name(cluster=w279, "Marker list"=w276) -> (w275:T2)
      n129 = property class="XYGraph (strict)"(reference=w280, "AnntList"=w276) -> ()  [unwired: 1 in, 2 out]
    }
    frame "MarkerStyle" {
      n130 = property class="XYGraph (strict)"(reference=w285) -> (reference out=w291:refnum<vi>, "AnntList"=w288:T6)  [unwired: 1 in, 1 out]
      n131 = Unbundle By Name(w290) -> ("Marker.Style"=w289:i32)
      n132 = for {
        tunnel: w289 -> [w294]
        tunnel: w288 -> [w293] mode=indexing
        tunnel: [w292] -> w287 mode=indexing
        n133 = Bundle By Name(cluster=w293, "Style"=w294) -> (w292:T12)
      }
      n134 = Bundle By Name(cluster=w290, "Marker list"=w287) -> (w286:T2)
      n135 = property class="XYGraph (strict)"(reference=w291, "AnntList"=w287) -> ()  [unwired: 1 in, 2 out]
    }
    frame "SelectorVisible" {
      w306 = T5[] [enum."Change Minimum Size"] items=["Update Polar Scale", "Cursor Release", "Autoscale", "Update Annotation", "Force Update Polar Scale", "Update Data", "Update Tree String", "Update Tree Checkbox", "Update Tree Opening", "Change Minimum Size"] ("operation in")
      n136 = Unbundle By Name(w303) -> ("Container bounds.Width"=w297:u32, "Container bounds.Height"=w296:u32)
      n137 = Bundle By Name(cluster=T7 {"Width"=0, "Height"=0} ("Previouse Container bounds"), "Width"=w297, "Height"=w296) -> (w295:T7)
      n138 = call <vilib>:"svx_Polar_Legend_Visible.vi"("Previous Container bounds"=w295, "Display State In"=w303, "z scale graph Refnum"=w299, "Plot Legend Refnum"=w300, "Polar Plot Refnum in"=w301, "Container Refnum"=w302) -> ("Display State out"=w304:T2)  [unwired: 1 in, 4 out]
      n139 = Build Array (concatenate)(w307, w306) -> (w305:T5[])
    }
    frame "Index" {
      w309 = T5[] [enum."Update Data", enum."Autoscale", enum."Update Polar Scale", enum."Cursor Release", enum."Update Annotation", enum."Update Tree String", enum."Update Tree Checkbox", enum."Update Tree Opening"] items=["Update Polar Scale", "Cursor Release", "Autoscale", "Update Annotation", "Force Update Polar Scale", "Update Data", "Update Tree String", "Update Tree Checkbox", "Update Tree Opening", "Change Minimum Size"]
    }
    frame "Legend Color" {
      w313 = -2 ("Active Cell:Active Column Number")
      n140 = Unbundle By Name(w312) -> ("Legend BG color"=w311:u32, "Legend font color"=w310:u32)
      n141 = property class="Tree (strict)"(reference=w314, "ActiveColNum"=w313, "Active Item Row Number"=w313, "CellBG"=w311, "CellFontColor"=w310) -> ()  [unwired: 1 in, 2 out]
    }
  }
  "operation out" <- w8
  "Display State Out" <- w6
